vi "Read Controls lib.vi"(8 "error in (no error)":errorcluster, 11 "BC-Panes in":refnum<class "MC-UI.lvclass">) -> (0 "error out":errorcluster, 2 "Controls lib":refnum<vi>[](array[refnum]), 3 "BC-Panes out":refnum<class "MC-UI.lvclass">)   [LabVIEW 2013, in "MaterialCharacterization.lvlib" / "MC-UI.lvclass"]
uses:
  MC-UI.lvclass
  MC-UI.lvclass/MC-UI.ctl
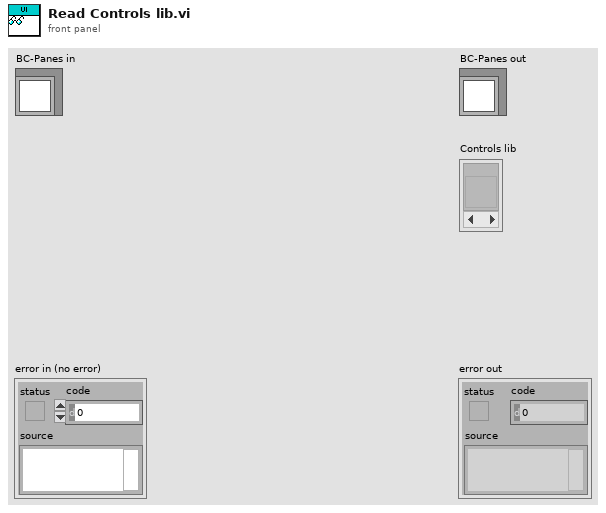
[diagram p1: front panel]
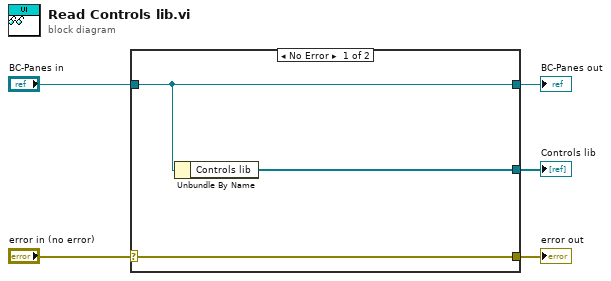
[diagram p0: block diagram]
diagram:
  n1 = case shown="No Error" "error in (no error)" {
    selector: "error in (no error)" -> [w8 w9]
    tunnel: [w8 w9] -> w4
    tunnel: [w7 w10] -> w2
    tunnel: "BC-Panes in" -> [w7 w10]
    tunnel: [w6 _] -> w1
    frame No Error {
      n2 = Unbundle By Name(w7) -> ("Controls lib"=w6:refnum<vi>[])
    }
    frame Error {
    }
  }
  "error out" <- w4
  "BC-Panes out" <- w2
  "Controls lib" <- w1
